vi "Theta Axis Control.vi"() -> ()   [LabVIEW 2017]
uses:
  <vilib>/myRIO/Express VI/Onboard IO/DO/DO Express VI.xnode
  <vilib>/myRIO/Instrument Drivers/Onboard IO/DIO/vis/Write.vi
  <vilib>/myRIO/Instrument Drivers/Onboard IO/DIO/DIO.lvlib
  <vilib>/myRIO/Common/Instrument Driver Framework/myRIO v1.0/DIO/typedefs/DIO Channels Enum.ctl
  <vilib>/myRIO/Common/Instrument Driver Framework/myRIO v1.0/DIO/typedefs/DIO Channels List.ctl
  <vilib>/myRIO/Common/Instrument Driver Framework/Utilities/typedefs/Generic FPGA Reference.ctl
  <vilib>/myRIO/Common/Instrument Driver Framework/Utilities/typedefs/myRIO v1.0 Reference.ctl
  <vilib>/myRIO/Common/Instrument Driver Framework/Utilities/typedefs/Hardware Version Enum.ctl
  <vilib>/myRIO/Common/Instrument Driver Framework/Utilities/typedefs/myRIO Generic Hardware Reference.ctl
  <vilib>/myRIO/Instrument Drivers/Onboard IO/DIO/typedefs/DIO Reference.ctl
  <vilib>/myRIO/Instrument Drivers/Onboard IO/DIO/vis/myRIO DIO Open.xnode
  <vilib>/myRIO/Common/Instrument Driver Framework/Utilities/vis/Is FPGA Ref Available.vi
  <vilib>/myRIO/Common/Instrument Driver Framework/myRIO v1.0/DIO/vis/myRIO v1.1 Open DIO.vi
  <vilib>/userdefined/High Color/nirio_resource_hc.ctl
panel:
  out "Boolean array":bool[](array[boolean])
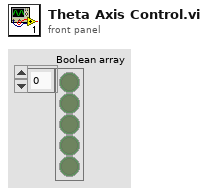
[diagram p1: front panel]
types:
  T1 = enum16{"Initialisation", "Step 1", "Step 2", "Step 3", "Step 4"}
  T2 = typedef "DIO.lvlib/DIO Reference.ctl" = cluster{"myRIO Reference":T3, "DIO Channels List":T7}
  T3 = typedef "myRIO Generic Hardware Reference.ctl" = cluster{"myRIO Model":T4, "myRIO Hardware Reference":T5}
  T4 = typedef "Hardware Version Enum.ctl" = enum16{"Unknown", "myRIO-1900", "myRIO-1950", "roboRIO", "NI ELVIS RIO CM"}
  T5 = typedef "myRIO v1.0 Reference.ctl" = cluster{"Generic FPGA Reference":T6, "Allow multiple opens":bool}
  T6 = typedef "Generic FPGA Reference.ctl" = refnum<k20>
  T7 = typedef "DIO Channels List.ctl" = T8[]
  T8 = typedef "DIO Channels Enum.ctl" = enum16{"Not Connected", "C/DIO0", "C/DIO1", "C/DIO2", "C/DIO3", "C/DIO4", "C/DIO5", "C/DIO6", "C/DIO7", "A/DIO0", "A/DIO1", "A/DIO2", "A/DIO3", "A/DIO4", "A/DIO5", "A/DIO6", "A/DIO7", "A/DIO8", "A/DIO9", "A/DIO10", "A/DIO11", "A/DIO12", "A/DIO13", "A/DIO14", "A/DIO15", "B/DIO0", "B/DIO1", "B/DIO2", "B/DIO3", "B/DIO4", "B/DIO5", "B/DIO6", "B/DIO7", "B/DIO8", "B/DIO9", "B/DIO10", "B/DIO11", "B/DIO12", "B/DIO13", "B/DIO14", "B/DIO15", "LED0", "LED1", "LED2", "LED3", "Button0", "DIO/DIO0", "DIO/DIO1", "DIO/DIO2", "DIO/DIO3", "DIO/DIO4", "DIO/DIO5", "DIO/DIO6", "DIO/DIO7", "DIO/DIO8", "DIO/DIO9", "SPI/CS0", "SPI/CS1", "SPI/CS2", "SPI/CS3", "LED RADIO (Green)", "LED RADIO (Red)", "LED COMM (Green)", "LED COMM (Red)", "LED MODE (Green)", "LED MODE (Red)"}
  T9 = typedef "nirio_resource_hc.ctl" = tag
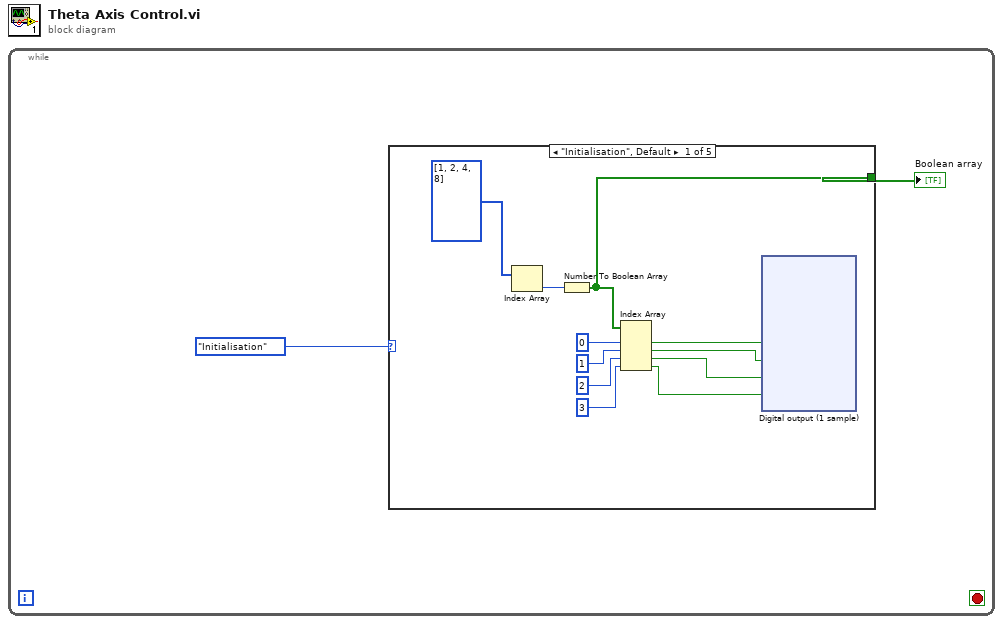
[diagram p0: block diagram]
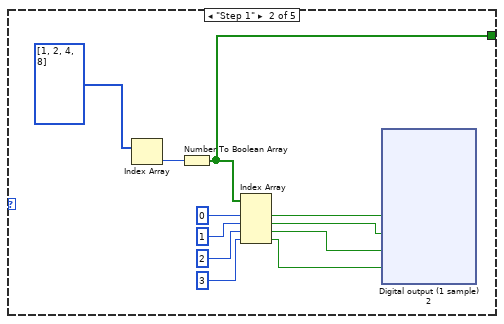
[diagram p2: hidden frame]
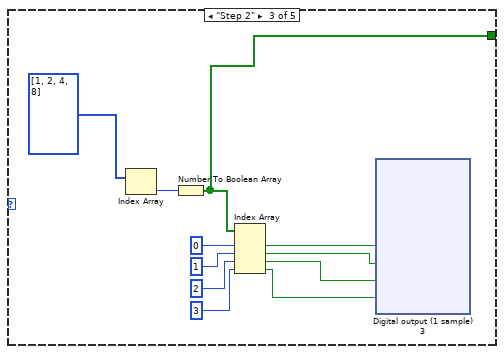
[diagram p3: hidden frame]
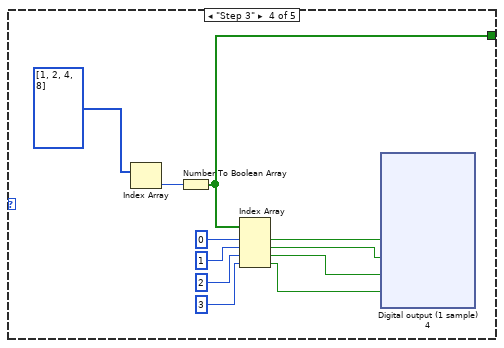
[diagram p4: hidden frame]
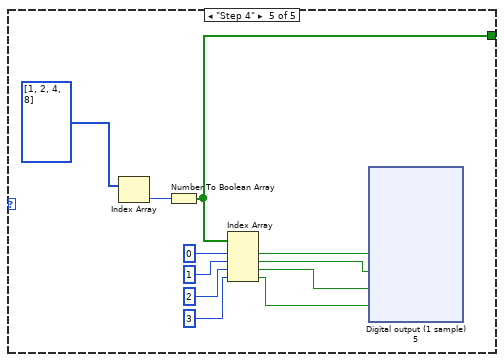
[diagram p5: hidden frame]
diagram:
  n1 = while {
    stop <- _ stop-if-true
    n2 = case shown="\"Initialisation\", Default" T1."Initialisation" {
      tunnel: [w5 w53 w101 w150 w199] -> w1
      frame "Initialisation", Default {
        n3 = Index Array(array=i32[] [1, 2, 4, 8]) -> (element=w4:i32)  [unwired: 1 in]
        n4 = Number To Boolean Array(number=w4) -> (Boolean array=w5:bool[])
        n5 = Index Array(array=w5, index #1=0 ("index"), index #2=1 ("index"), index #3=2 ("index"), index #4=3 ("index")) -> (element #1=w13:bool, element #2=w12:bool, element #3=w11:bool, element #4=w10:bool)
        n6 = xnode "Digital output (1 sample)"("A/DIO0 (Pin 11)"=w13, "A/DIO1 (Pin 13)"=w12, "A/DIO2 (Pin 15)"=w11, "A/DIO3 (Pin 17)"=w10) -> ()  [unwired: 1 in, 1 out]
      }
      frame "Step 1" {
        n7 = Index Array(array=i32[] [1, 2, 4, 8]) -> (element=w54:i32)  [unwired: 1 in]
        n8 = Number To Boolean Array(number=w54) -> (Boolean array=w53:bool[])
        n9 = Index Array(array=w53, index #1=0 ("index"), index #2=1 ("index"), index #3=2 ("index"), index #4=3 ("index")) -> (element #1=w62:bool, element #2=w61:bool, element #3=w60:bool, element #4=w59:bool)
        n10 = xnode "Digital output (1 sample) 2"("A/DIO0 (Pin 11)"=w62, "A/DIO1 (Pin 13)"=w61, "A/DIO2 (Pin 15)"=w60, "A/DIO3 (Pin 17)"=w59) -> ()  [unwired: 1 in, 1 out]
      }
      frame "Step 2" {
        n11 = Index Array(array=i32[] [1, 2, 4, 8]) -> (element=w103:i32)  [unwired: 1 in]
        n12 = Number To Boolean Array(number=w103) -> (Boolean array=w101:bool[])
        n13 = Index Array(array=w101, index #1=0 ("index"), index #2=1 ("index"), index #3=2 ("index"), index #4=3 ("index")) -> (element #1=w111:bool, element #2=w110:bool, element #3=w109:bool, element #4=w108:bool)
        n14 = xnode "Digital output (1 sample) 3"("A/DIO0 (Pin 11)"=w111, "A/DIO1 (Pin 13)"=w110, "A/DIO2 (Pin 15)"=w109, "A/DIO3 (Pin 17)"=w108) -> ()  [unwired: 1 in, 1 out]
      }
      frame "Step 3" {
        n15 = Index Array(array=i32[] [1, 2, 4, 8]) -> (element=w152:i32)  [unwired: 1 in]
        n16 = Number To Boolean Array(number=w152) -> (Boolean array=w150:bool[])
        n17 = Index Array(array=w150, index #1=0 ("index"), index #2=1 ("index"), index #3=2 ("index"), index #4=3 ("index")) -> (element #1=w160:bool, element #2=w159:bool, element #3=w158:bool, element #4=w157:bool)
        n18 = xnode "Digital output (1 sample) 4"("A/DIO0 (Pin 11)"=w160, "A/DIO1 (Pin 13)"=w159, "A/DIO2 (Pin 15)"=w158, "A/DIO3 (Pin 17)"=w157) -> ()  [unwired: 1 in, 1 out]
      }
      frame "Step 4" {
        n19 = Index Array(array=i32[] [1, 2, 4, 8]) -> (element=w201:i32)  [unwired: 1 in]
        n20 = Number To Boolean Array(number=w201) -> (Boolean array=w199:bool[])
        n21 = Index Array(array=w199, index #1=0 ("index"), index #2=1 ("index"), index #3=2 ("index"), index #4=3 ("index")) -> (element #1=w209:bool, element #2=w208:bool, element #3=w207:bool, element #4=w206:bool)
        n22 = xnode "Digital output (1 sample) 5"("A/DIO0 (Pin 11)"=w209, "A/DIO1 (Pin 13)"=w208, "A/DIO2 (Pin 15)"=w207, "A/DIO3 (Pin 17)"=w206) -> ()  [unwired: 1 in, 1 out]
      }
    }
    "Boolean array" <- w1
  }
